vi "Create DVR.vi"(8 "error in (no error)":errorcluster, 11 "LogicIO in":refnum<class "LogicIO.lvclass">) -> (0 "error out":errorcluster, 2 "data value reference":refnum<data-value>, 3 "LogicIO out":refnum<class "LogicIO.lvclass">)   [LabVIEW 2016, in "Hardware.lvlib" / "LogicIO.lvlib" / "LogicIO.lvclass"]
uses:
  <userlib>/Common Components/Hardware/LogicIO/LogicIO/LogicIO.lvclass
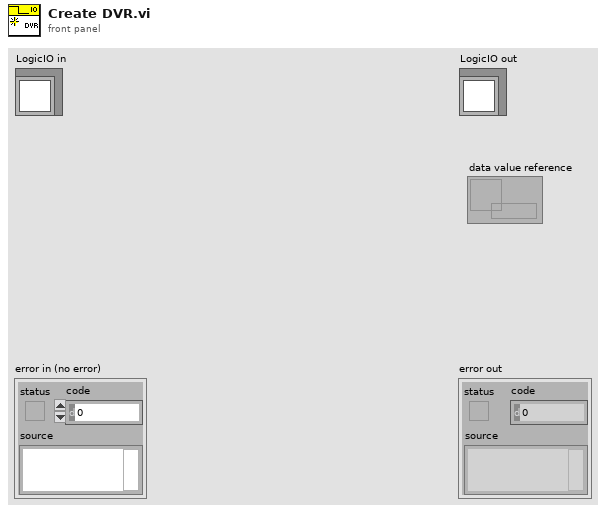
[diagram p1: front panel]
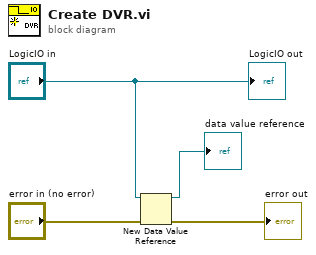
[diagram p0: block diagram]
diagram:
  n1 = New Data Value Reference(data value="LogicIO in", error in="error in (no error)") -> (data value reference=→"data value reference":refnum<data-value>, error out=→"error out":errorcluster)
  "LogicIO out" <- "LogicIO in"
